vi "Decode.vi"(8 "error in (no error)":errorcluster, 11 "data":waveform(dbl)[](array[waveform])) -> (0 "error out":errorcluster, 3 "Array":u8[](array[numeric]))   [LabVIEW 2018]
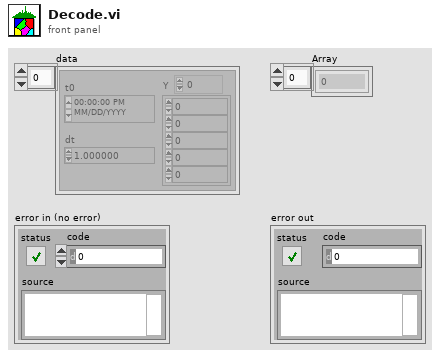
[diagram p1: front panel]
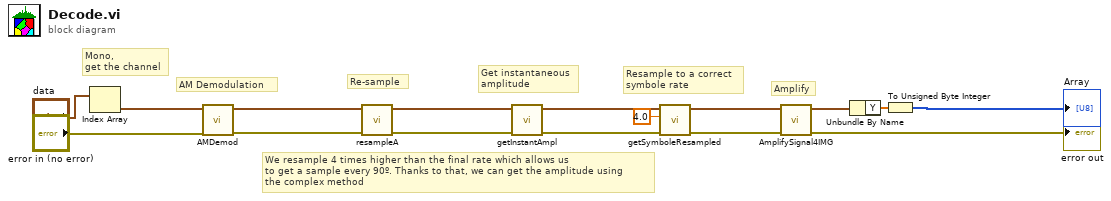
[diagram p0: block diagram]
diagram:
  # "We resample 4 times higher than the final rate which allows us\nto get a sample every 90º. Thanks to that, we can get the amplitude using\nthe complex method"
  # "Amplify"
  # "Mono,\nget the channel"
  # "Resample to a correct\nsymbole rate"
  # "Get instantaneous\namplitude"
  # "Re-sample"
  # "AM Demodulation"
  n1 = Index Array(array="data") -> (element=w2:waveform(dbl))  [unwired: 1 in]
  n2 = call "AMDemod.vi"("error in (no error)"="error in (no error)", "data"=w2) -> ("error out"=w9:errorcluster, "Waveform"=w3:waveform(dbl))  [unwired: 8 in]
  n3 = call "resampleA.vi"("error in (no error)"=w9, "Waveform"=w3) -> ("error out"=w10:errorcluster, "resampled waveform out"=w4:waveform(dbl))  [unwired: 8 in]
  n4 = call "getInstantAmpl.vi"("error in (no error)"=w10, "resampled waveform in"=w4) -> ("error out"=w11:errorcluster, "Waveform"=w5:waveform(dbl))  [unwired: 8 in]
  n5 = call "getSymboleResampled.vi"("error in (no error)"=w11, "Multiplier"=4.0, "Waveform"=w5) -> ("error out"=w13:errorcluster, "resampled waveform out"=w6:waveform(dbl))  [unwired: 7 in]
  n6 = call "AmplifySignal4IMG.vi"("error in (no error)"=w13, "resampled waveform in"=w6) -> ("error out"=→"error out":errorcluster, "Waveform"=w7:waveform(dbl))  [unwired: 8 in]
  n7 = Unbundle By Name(w7) -> ("Y"=w8:dbl[])
  n8 = To Unsigned Byte Integer(number=w8) -> (unsigned 8bit integer=→"Array":u8[])
